vi "Analyze Response.vi"(8 "error in (no error)":errorcluster, 10 "body":string, 11 "headers":string) -> (0 "error out":errorcluster)   [LabVIEW 2015, in "PL eLabFTW Client.lvclass"]
doc: "Analyzes HTTP response and returns error if status code is not 200."
uses:
  PL eLabFTW Client.lvclass
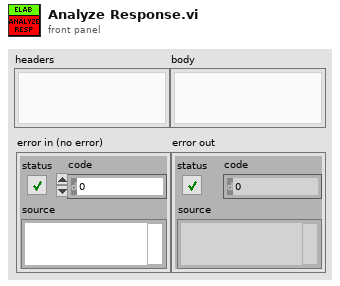
[diagram p1: front panel]
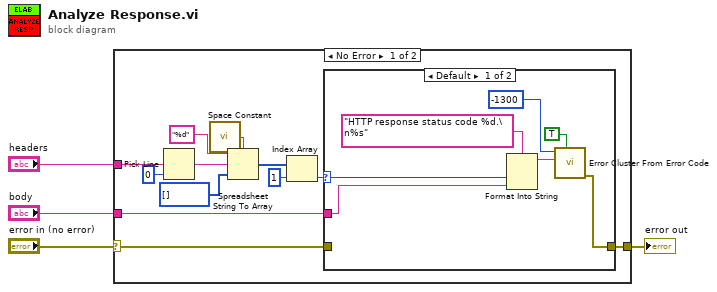
[diagram p0: block diagram]
diagram:
  n1 = case shown="No Error" "error in (no error)" {
    selector: "error in (no error)" -> [w7 w25]
    tunnel: [w6 w25] -> w3
    tunnel: "headers" -> [w16 _]
    tunnel: "body" -> [w5 _]
    frame No Error {
      n2 = Pick Line(multi-line string=w16, line index=0) -> (output string=w13:string)  [unwired: 1 in]
      n3 = call <vilib>:"Space Constant.vi"() -> ("String"=w11:string)
      n4 = Spreadsheet String To Array(delimiter (Tab)=w11, format string="%d", spreadsheet string=w13, array type (2D Dbl)=i32[] []) -> (array=w10:i32[])
      n5 = Index Array(array=w10, index=1) -> (element=w8:i32)
      n6 = case shown="Default" w8 {
        selector: w8 -> [w19 _]
        tunnel: w7 -> [_ w24]
        tunnel: [w18 w24] -> w6
        tunnel: w5 -> [w17 _]
        frame Default {
          n7 = Format Into String(format string="HTTP response status code %d.\n%s", w19, w17) -> (resulting string=w20:string)  [unwired: 2 in, 1 out]
          n8 = call <vilib>:"Error Cluster From Error Code.vi"("show call chain? (False)"=TRUE, "error message (\"\")"=w20, "error code (0)"=-1300) -> ("error out"=w18:errorcluster)  [unwired: 6 in]
        }
        frame 200 {
        }
      }
    }
    frame Error {
    }
  }
  "error out" <- w3
